vi "Display Brightness (Set).vi"(6 "ISOBUS address":T3=-1 caption="ISOBUS address (-1)", 8 "error in":errorcluster, 10 "Display Brightness":string, 11 "Mercury Reference In":T4) -> (0 "error out":errorcluster, 2 "Response":T2, 3 "Mercury Reference Out":T4, 4 "Valid?":T1)   [LabVIEW 2014, in "Mercury iXX.lvlib" / "System.lvlib"]
doc: "Set the display brightness of the instrument."
uses:
  System.lvlib
  Controls/Mercury Reference.ctl
  Controls/Comms Transport Layer.ctl
  Private/Controls/Query Dynamic Reference.ctl
  Controls/ISOBus Address.ctl
  Controls/Response String.ctl
  Controls/Is Valid LED.ctl
  Private/Controls/Command Verbs.ctl
  Mercury iXX.lvlib
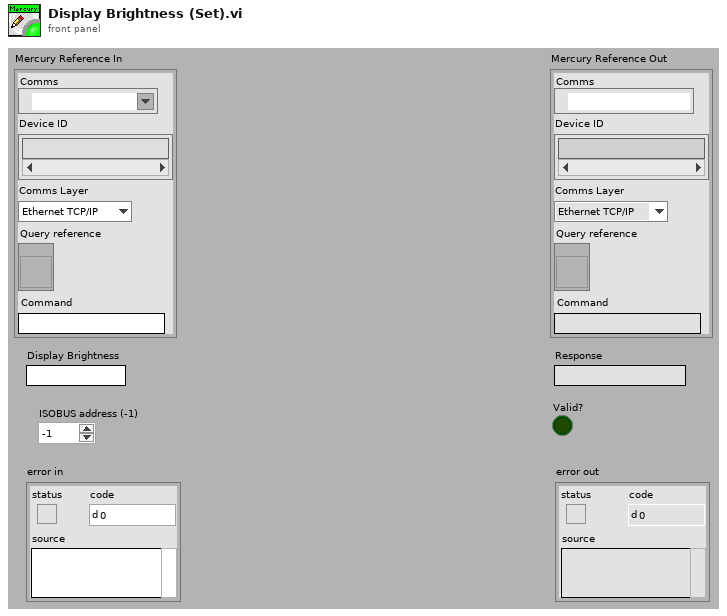
[diagram p1: front panel]
types:
  T1 = typedef "Mercury iXX.lvlib/Is Valid LED.ctl" = bool
  T2 = typedef "Mercury iXX.lvlib/Response String.ctl" = string
  T3 = typedef "Mercury iXX.lvlib/ISOBus Address.ctl" = i32
  T4 = typedef "Mercury iXX.lvlib/Mercury Reference.ctl" = cluster{"Comms":refnum<visa-resource-name>, "Device ID":string[], "Comms Layer":T5, "Command":string, "Query reference":T6}
  T5 = typedef "Mercury iXX.lvlib/Comms Transport Layer.ctl" = enum16{"Ethernet TCP/IP", "USB", "ISOBus - RS-232", "GPIB"}
  T6 = typedef "Mercury iXX.lvlib/Query Dynamic Reference.ctl" = refnum<vi>
  T7 = typedef "Mercury iXX.lvlib/Command Verbs.ctl" = string
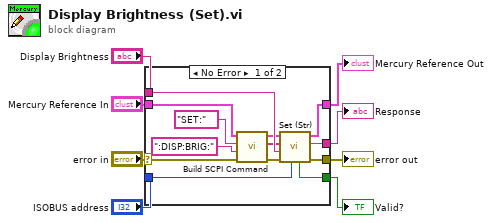
[diagram p0: block diagram]
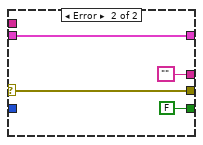
[diagram p2: hidden frame]
diagram:
  n1 = case shown="No Error" "error in" {
    selector: "error in" -> [w9 w24]
    tunnel: "Mercury Reference In" -> [w13 w25]
    tunnel: [w15 w25] -> w7
    tunnel: [w19 w24] -> w6
    tunnel: "ISOBUS address" -> [w17 _]
    tunnel: [w16 ""] -> w3
    tunnel: "Display Brightness" -> [w20 _]
    tunnel: [w18 FALSE ("Valid?")] -> w1
    frame No Error {
      n2 = call "Build SCPI Command.vi"("error in"=w9, "Noun(s)"=":DISP:BRIG:" ("Command"), "Verb"=T7 "SET:", "Mercury Reference In"=w13) -> ("error out"=w11:errorcluster, "SCPI Message(s)"=w10:string[], "Mercury Reference Out"=w12:T4)  [unwired: 5 out]
      n3 = call "Set (Str).vi"("ISOBUS address"=w17, "error in"=w11, "Command Value (Str)"=w20, "SCPI Message(s)"=w10, "Mercury Reference In"=w12) -> ("error out"=w19:errorcluster, "Response"=w16:T2, "Mercury Reference Out"=w15:T4, "Valid?"=w18:T1)  [unwired: 3 out]
    }
    frame Error {
    }
  }
  "Mercury Reference Out" <- w7
  "error out" <- w6
  "Response" <- w3
  "Valid?" <- w1
